vi "New User.vi"(8 "error in (no error)":errorcluster, 10 "userinfo":T1, 11 "[User] Userinfo Binary in":refnum<class "[User] Userinfo Binary.lvclass">) -> (0 "error out":errorcluster, 3 "[User] Userinfo Binary out":refnum<class "[User] Userinfo Binary.lvclass">)   [LabVIEW 2020, in "[User] Userinfo Binary.lvclass"]
uses:
  [User] Userinfo Binary.lvclass
  [User] Userinfo/Control/userinfo.ctl
  [User] Userinfo Binary.lvclass/[User] Userinfo Binary.ctl
  [User] Userinfo/[User] Userinfo.lvclass
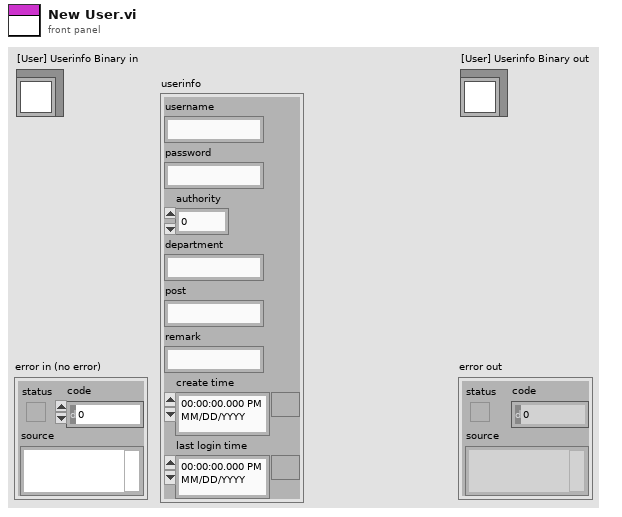
[diagram p1: front panel]
types:
  T1 = typedef "[User] Userinfo.lvclass/userinfo.ctl" = cluster{"username":string, "password":string, "authority":i8, "department":string, "post":string, "remark":string, "create time":timestamp, "last login time":timestamp}
  T2 = cluster{"password":string, "authority":i8, "department":string, "post":string, "remark":string, "create time":timestamp, "last login time":timestamp}
  T3 = typedef "[User] Userinfo Binary.lvclass/userinfo.ctl" = cluster{"password":string, "authority":i8, "department":string, "post":string, "remark":string, "create time":timestamp, "last login time":timestamp}
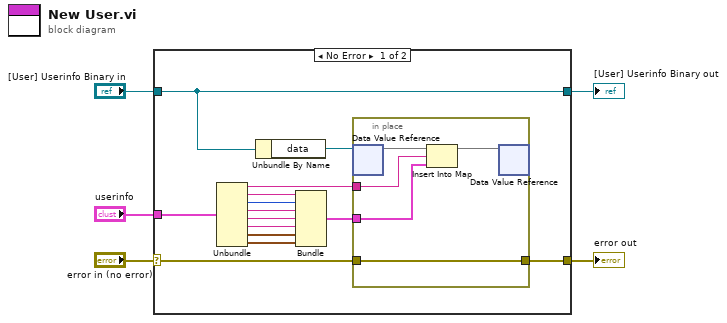
[diagram p0: block diagram]
diagram:
  n1 = case shown="No Error" "error in (no error)" {
    selector: "error in (no error)" -> [w10 w26]
    tunnel: [w6 w26] -> w3
    tunnel: "[User] Userinfo Binary in" -> [w9 w25]
    tunnel: [w9 w25] -> w1
    tunnel: "userinfo" -> [w11 _]
    frame No Error {
      n2 = Unbundle(w11) -> ("username"=w12:string, "password"=w15:string, "authority"=w16:i8, "department"=w17:string, "post"=w18:string, "remark"=w19:string, "create time"=w8:timestamp, "last login time"=w7:timestamp)
      n3 = Unbundle By Name(w9) -> ("data"=w14:refnum<data-value>)
      n4 = Bundle("password"=w15, "authority"=w16, "department"=w17, "post"=w18, "remark"=w19, "create time"=w8, "last login time"=w7) -> (w13:T2)  [unwired: 1 in]
      n5 = in-place {
        in-place-border: w13 -> [w22]
        in-place-border: w12 -> [w23]
        in-place-border: w10 -> [w20]
        in-place-border: [w20] -> w6
        n6 = in-place-dvr #1(w14) -> (w24:map{string, T3})  [unwired: 1 out]
        n7 = Insert Into Map(map in=w24, key=w23, value=w22) -> (map out=w21:map{string, T3})  [unwired: 2 out]
        n8 = in-place-dvr #1(w21) -> ()  [unwired: 2 out]
      }
    }
    frame Error {
    }
  }
  "error out" <- w3
  "[User] Userinfo Binary out" <- w1
